vi "Configure_1GHz clock.vi"(8 "error in":errorcluster, 11 "FPGA SPI config ref":T1) -> (0 "error out":errorcluster, 3 "FPGA SPI config out":T1)   [LabVIEW 2013]
uses:
  SPI config/FPGA_spi_config.ctl
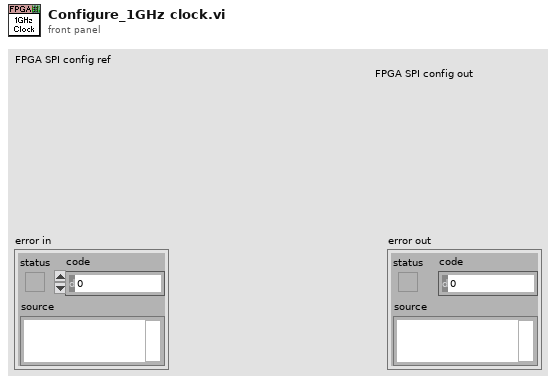
[diagram p1: front panel]
types:
  T1 = typedef "FPGA_spi_config.ctl" = refnum<k20>
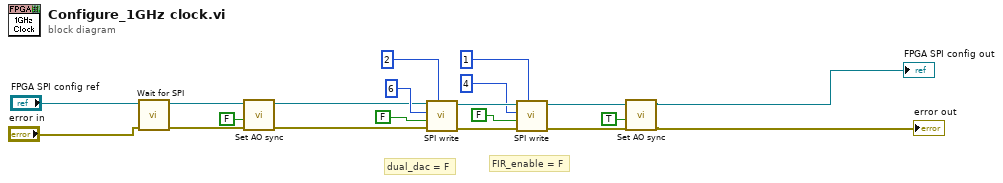
[diagram p0: block diagram]
diagram:
  # "FIR_enable = F"
  # "dual_dac = F"
  n1 = call "Wait for SPI.vi"("error in"="error in", "FPGA SPI config ref"="FPGA SPI config ref") -> ("error out"=w1:errorcluster, "FPGA SPI config out"=w3:T1)  [unwired: 7 in, 1 out]
  n2 = call "Set AO sync.vi"("error in"=w1, "AO sync"=FALSE, "FPGA SPI config ref"=w3) -> ("error out"=w9:errorcluster, "FPGA SPI config out"=w10:T1)  [unwired: 7 in]
  n3 = call "SPI write.vi"("SPI Address"=u16 2, "error in"=w9, "Value"=FALSE, "Bit"=u16 6, "FPGA SPI config ref"=w10) -> ("error out"=w15:errorcluster, "FPGA SPI config out"=w16:T1)  [unwired: 5 in]
  n4 = call "SPI write.vi"("SPI Address"=u16 1, "error in"=w15, "Value"=FALSE, "Bit"=u16 4, "FPGA SPI config ref"=w16) -> ("error out"=w8:errorcluster, "FPGA SPI config out"=w11:T1)  [unwired: 5 in]
  n5 = call "Set AO sync.vi"("error in"=w8, "AO sync"=TRUE, "FPGA SPI config ref"=w11) -> ("error out"=→"error out":errorcluster, "FPGA SPI config out"=→"FPGA SPI config out":T1)  [unwired: 7 in]
